vi "TabOver.vi"(11 "Array in":string[](array[string])) -> (3 "Array out":string[](array[string]))   [LabVIEW 2017]
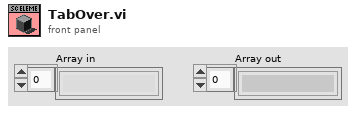
[diagram p1: front panel]
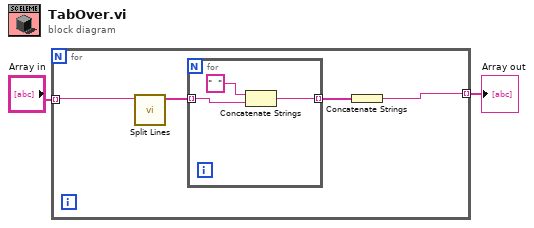
[diagram p0: block diagram]
diagram:
  n1 = for {
    tunnel: "Array in" -> [w6] mode=indexing
    tunnel: [w3] -> w2 mode=indexing
    n2 = call "Split Lines.vi"("String"=w6) -> ("Array"=w5:string[])  [unwired: 10 in]
    n3 = for {
      tunnel: w5 -> [w7] mode=indexing
      tunnel: [w8] -> w4 mode=indexing
      n4 = Concatenate Strings("  ", w7) -> (w8:string)
    }
    n5 = Concatenate Strings(w4) -> (w3:string)
  }
  "Array out" <- w2
